vi "_builtins_rect_map.vi"(9 "Values":variant[](array[variant]), 10 "Is Indicator?":bool[](array[boolean]), 11 "Rects in":T1[](array[typedef])) -> (1 "Row Heights":i16[](array[numeric]), 2 "Column Widths":i16[](array[numeric]), 3 "2D Index Map out":i32[][](array[numeric]))   [LabVIEW 2019, in "Script.lvlib"]
doc: "Resolves the front panel control map using the control bounds and values to align same types."
uses:
  Script.lvlib
  <vilib>/Utility/miscctls.llb/LVRectTypeDef.ctl
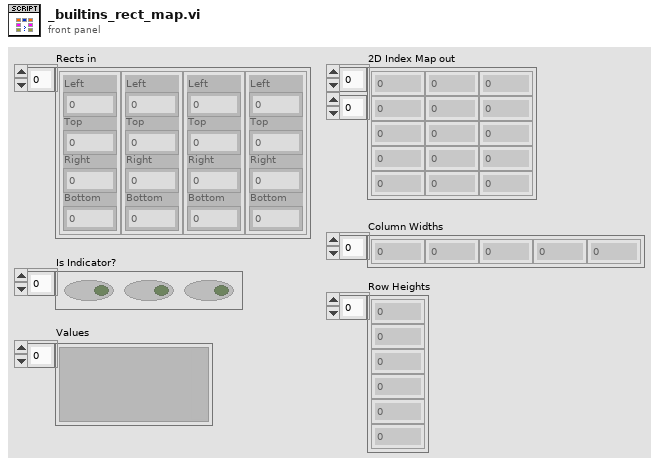
[diagram p1: front panel]
types:
  T1 = typedef "LVRectTypeDef.ctl" = cluster{"Left":i16, "Top":i16, "Right":i16, "Bottom":i16}
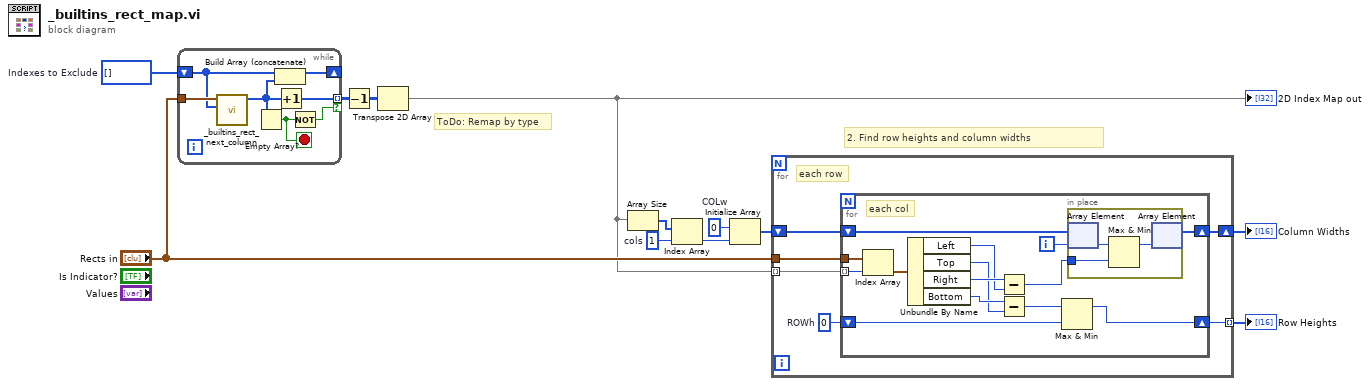
[diagram p0: block diagram]
diagram:
  w5 = i32[] []  # Indexes to Exclude
  w9 = i16 0  # COLw
  w10 = 1  # cols
  # "ToDo: Remap by type"
  # "2. Find row heights and column widths"
  n1 = while {
    tunnel: "Rects in" -> [w19]
    tunnel: [w18] -> w3 mode=indexing if=w13
    shift-right: [w15] -> _
    shift-left: w5 -> [w17]
    stop <- w14 stop-if-true
    n2 = call "_builtins_rect_next_column.vi"("Indexes to Exclude"=w17, "Rects in"=w19) -> ("Next Column Indexes"=w16:i32[])  [unwired: 9 in]
    n3 = Empty Array?(array=w16) -> (empty?=w14:bool)
    n4 = Build Array (concatenate)(w17, w16) -> (w15:i32[])
    n5 = Increment(x=w16) -> (x+1=w18:i32[])
    n6 = Not(x=w14) -> (.not. x?=w13:bool)
  }
  n7 = Decrement(x=w3) -> (x-1=w2:i32[][])
  n8 = Transpose 2D Array(2D array=w2) -> (transposed array=w1:i32[][])
  "2D Index Map out" <- w1
  n9 = Array Size(array=w1) -> (size(s)=w12:i32[])
  n10 = Index Array(array=w12, index=w10) -> (element=w11:i32)
  n11 = Initialize Array(w9, w11) -> (w8:i16[])
  n12 = for {
    tunnel: w1 -> [w24] mode=indexing
    tunnel: "Rects in" -> [w25]
    tunnel: [w22] -> w6 mode=indexing
    shift-right: [w21] -> w7
    shift-left: w8 -> [w20]
    w23 = i16 0  # ROWh
    # "each row"
    n13 = for {
      tunnel: w25 -> [w39]
      tunnel: w24 -> [w38] mode=indexing
      shift-right: [w31] -> w22
      shift-left: w23 -> [w32]
      shift-right: [w28] -> w21
      shift-left: w20 -> [w27]
      i -> [w26]
      # "each col"
      n14 = Index Array(array=w39, index=w38) -> (element=w37:T1)
      n15 = Unbundle By Name(w37) -> ("Left"=w35:i16, "Top"=w33:i16, "Right"=w36:i16, "Bottom"=w34:i16)
      n16 = Subtract(x=w36, y=w35) -> (x-y=w29:i16)
      n17 = Subtract(x=w34, y=w33) -> (x-y=w30:i16)
      n18 = Max & Min(x=w30, y=w32) -> (max(x,y)=w31:i16)  [unwired: 1 out]
      n19 = in-place {
        in-place-border: w29 -> [w41]
        n20 = in-place-array #1(w27, w26) -> (w42:i16)
        n21 = Max & Min(x=w42, y=w41) -> (max(x,y)=w40:i16)  [unwired: 1 out]
        n22 = in-place-array #1(w40) -> (w28:i16[])  [unwired: 1 out]
      }
    }
  }
  "Column Widths" <- w7
  "Row Heights" <- w6
